vi "StateEstimator.vi"(0 "latitude position degrees":dbl, 1 "longitude position degrees":dbl, 2 "GPS - km/h":string, 3 "GPS - Psi":string, 4 "IMU GYRO":cluster{dbl, dbl, dbl}, 5 "IMU ACC":cluster{dbl, dbl, dbl}, 6 "Steering position (counts)":i32, 7 "error in (no error)":errorcluster, 8 "Time step (s)":dbl) -> (14 "error out":errorcluster, 15 "Estimated position X (m)":dbl, 16 "Estimated position Y (m)":dbl, 17 "Estimated track angle Psi (rad)":dbl, 18 "Estimated roll (rad)":dbl, 19 "Estimated roll rate (rad/s)":dbl)   [LabVIEW 2019]
uses:
  libstate_estimator.dll
  <vilib>/LabVIEW Open Source Project/Data Manipulation/Scalar/OpenScalar.lvlib
  <vilib>/Utility/file.llb/Write Delimited Spreadsheet (string).vi
panel:
  out "latitude position rad":dbl
  out "longitude position rad":dbl
  out "Steering angle (radians)":dbl
  out "IMU ACC (Z) m/s2":dbl
  out "IMU ACC (Y) m/s2":dbl
  out "IMU ACC (X) m/s2":dbl
  out "IMU yaw rate (Z) rad/s":dbl
  out "IMU pitch rate (Y) rad/s":dbl
  out "IMU roll rate (X) rad/s":dbl
  out "GPS - Psi (rad)":dbl format="%#.6f"
  out "GPS - velocity (m/s)":dbl format="%#.6f"
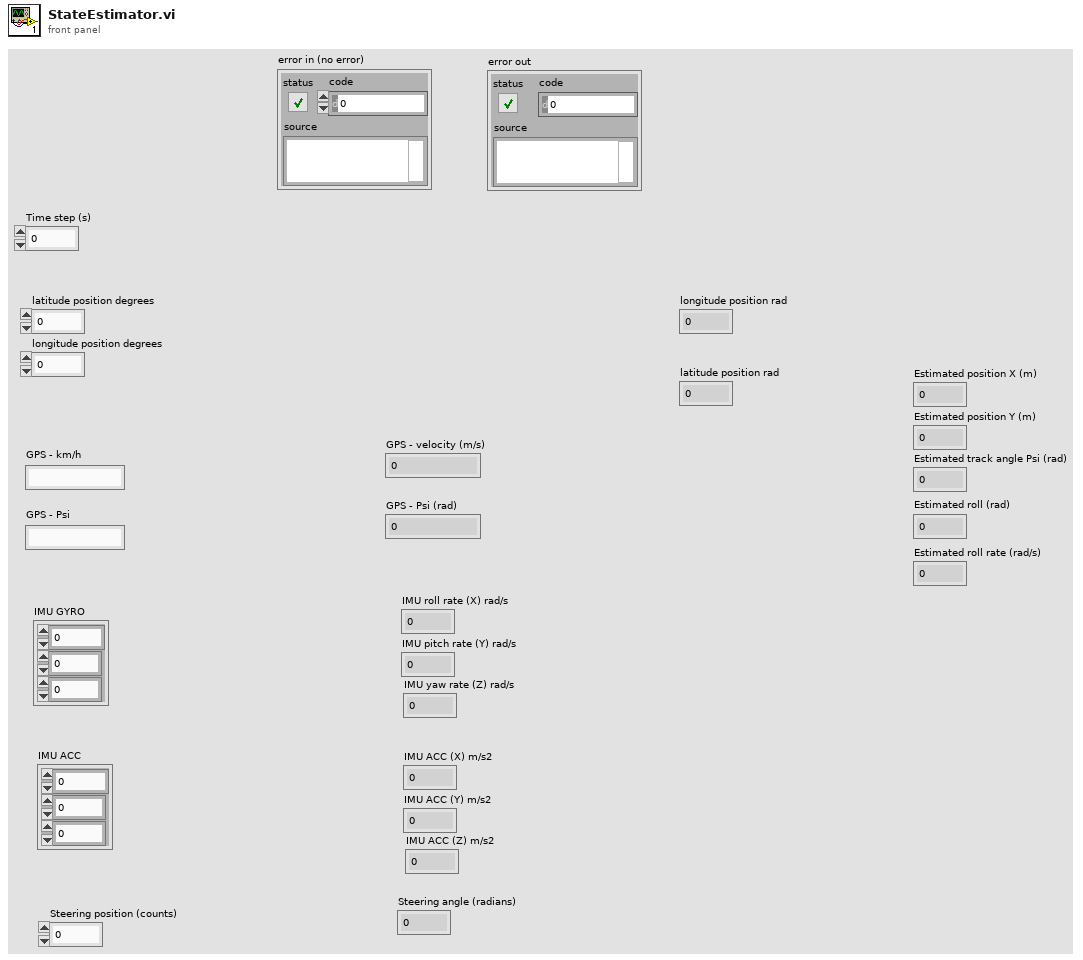
[diagram p1: front panel]
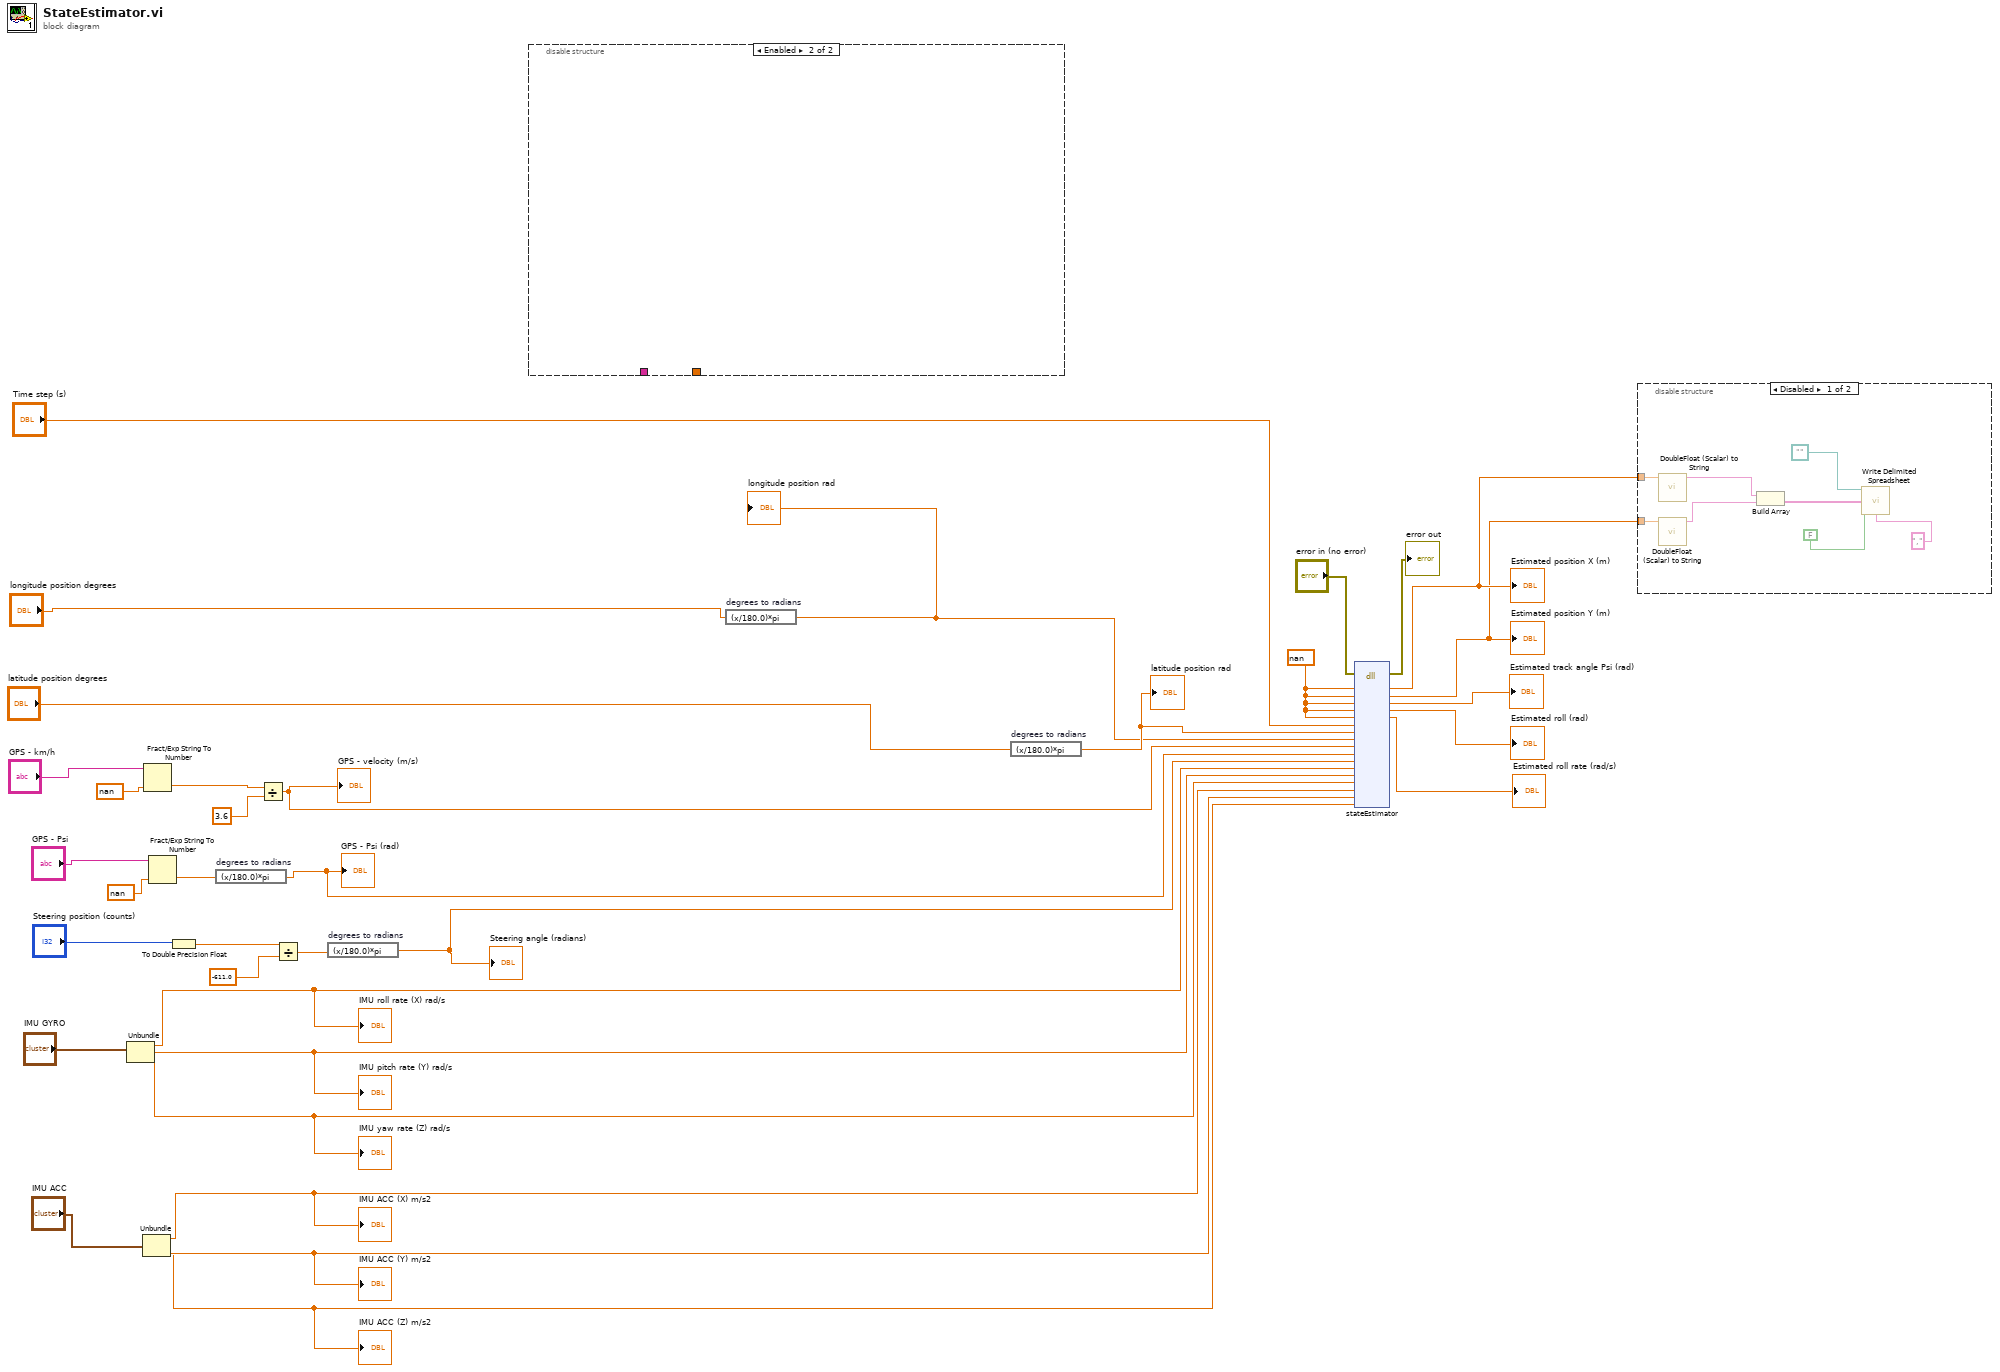
[diagram p0: block diagram]
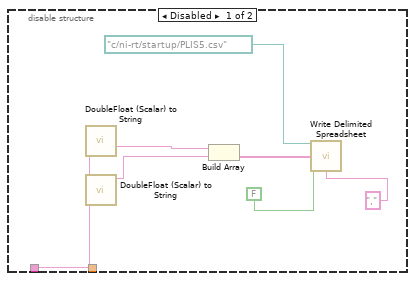
[diagram p2: hidden frame]
diagram:
  w22 = nan
  n1 = Unbundle("IMU GYRO") -> (w9:dbl, w8:dbl, w4:dbl)
  "IMU roll rate (X) rad/s" <- w9
  "IMU pitch rate (Y) rad/s" <- w8
  "IMU yaw rate (Z) rad/s" <- w4
  n2 = Unbundle("IMU ACC") -> (w6:dbl, w7:dbl, w5:dbl)
  "IMU ACC (X) m/s2" <- w6
  "IMU ACC (Y) m/s2" <- w7
  "IMU ACC (Z) m/s2" <- w5
  n3 = Fract/Exp String To Number(string="GPS - km/h", default (0 dbl)=nan) -> (number=w31:dbl)  [unwired: 2 in, 1 out]
  n4 = Fract/Exp String To Number(string="GPS - Psi", default (0 dbl)=nan) -> (number=w29:dbl)  [unwired: 2 in, 1 out]
  n5 = To Double Precision Float(number="Steering position (counts)") -> (double precision float=w26:dbl)
  n6 = expression code="(x/180.0)*pi" "degrees to radians"(w29) -> (w10:dbl)
  "GPS - Psi (rad)" <- w10
  n7 = Divide(x=w31, y=3.6) -> (x/y=w3:dbl)
  "GPS - velocity (m/s)" <- w3
  n8 = Divide(x=w26, y=-611.0) -> (x/y=w25:dbl)
  n9 = expression code="(x/180.0)*pi" "degrees to radians"(w25) -> (w12:dbl)
  "Steering angle (radians)" <- w12
  n10 = disable-structure shown="Enabled" {
    disable-tunnel: _ -> [w43 _]
    disable-tunnel: _ -> [w42 _]
    frame Disabled {
      n11 = call <vilib>:"DoubleFloat (Scalar) to String.vi"("Value (Double)"=w43) -> ("Value (String)"=w36:string)  [unwired: 10 in]
      n12 = call <vilib>:"DoubleFloat (Scalar) to String.vi"("Value (Double)"=w42) -> ("Value (String)"=w41:string)  [unwired: 10 in]
      n13 = Build Array(w36, w41) -> (w38:string[])
      n14 = call-poly <vilib>:"Write Delimited Spreadsheet.vi"("file path (dialog if empty)"=path "c:/ni-rt/startup/PLIS5.csv", "1D data"=w38, "append to file? (new file:F)"=FALSE, "delimiter (\\t)"="," ("delimiter (\\t)")) -> ()  [unwired: 10 in, 2 out]
    }
    frame Enabled {
    }
  }
  n15 = expression code="(x/180.0)*pi" "degrees to radians"("longitude position degrees") -> (w20:dbl)
  "longitude position rad" <- w20
  n16 = expression code="(x/180.0)*pi" "degrees to radians"("latitude position degrees") -> (w21:dbl)
  "latitude position rad" <- w21
  n17 = dll-call lib="libstate_estimator.*" fn="stateEstimator"(error in="error in (no error)", "X"=w22, "Y"=w22, "Psi"=w22, "roll"=w22, "rollRate"=w22, "Ts"="Time step (s)", "latitude"=w21, "longitude"=w20, "speed"=w3, "headingAngle"=w10, "steeringAngle"=w12, "gyroX"=w9, "gyroY"=w8, "gyroZ"=w4, "accX"=w6, "accY"=w7, "accZ"=w5) -> (error out=→"error out":errorcluster, "X"=w14:dbl, "Y"=w13:dbl, "Psi"=→"Estimated track angle Psi (rad)":dbl, "roll"=→"Estimated roll (rad)":dbl, "rollRate"=→"Estimated roll rate (rad/s)":dbl)  [unwired: 15 in, 1 out]
  "Estimated position X (m)" <- w14
  "Estimated position Y (m)" <- w13
  n18 = disable-structure shown="Disabled" {
    disable-tunnel: w14 -> [w45 _]
    disable-tunnel: w13 -> [w44 _]
    frame Disabled {
      n19 = call <vilib>:"DoubleFloat (Scalar) to String.vi"("Value (Double)"=w45) -> ("Value (String)"=w51:string)  [unwired: 10 in]
      n20 = call <vilib>:"DoubleFloat (Scalar) to String.vi"("Value (Double)"=w44) -> ("Value (String)"=w50:string)  [unwired: 10 in]
      n21 = Build Array(w51, w50) -> (w47:string[])
      n22 = call-poly <vilib>:"Write Delimited Spreadsheet.vi"("file path (dialog if empty)"=path "", "1D data"=w47, "append to file? (new file:F)"=FALSE, "delimiter (\\t)"="," ("delimiter (\\t)")) -> ()  [unwired: 10 in, 2 out]
    }
    frame Enabled {
    }
  }
